vi "AlliGator Check Calibration Menu Items.vi"(8 "Use Calibration Phasor Map":bool, 9 "Use Calibration Phasor Curve":bool, 10 "Use Calibration Phasor":bool, 11 "Menu in":refnum<k9>) -> (3 "menu reference out":refnum<k9>)   [LabVIEW 2021, in "AlliGator Phasor Calibration.lvlib"]
doc: "Checks the appropriate menu item telling what type of calibration is used (single phasor, map or series)."
uses:
  AlliGator Phasor Calibration.lvlib
panel:
  # "see the AlliGator License on the block diagram (Ctrl+E or Window:Show Block Diagram)"
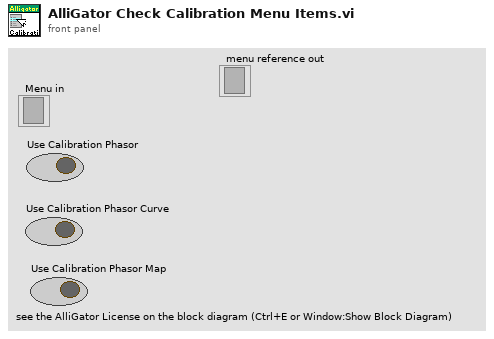
[diagram p1: front panel]
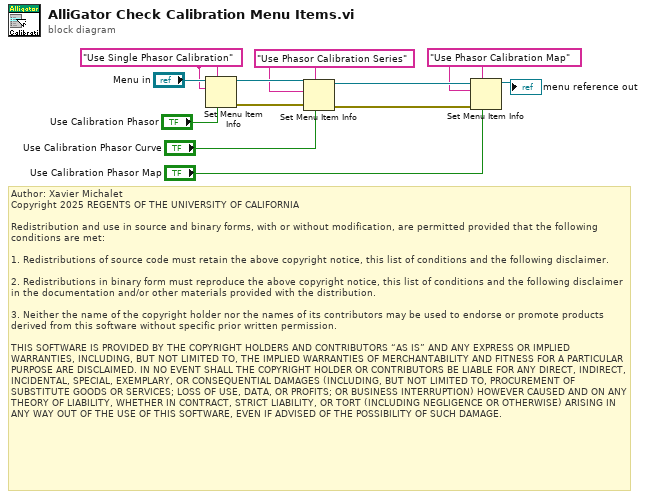
[diagram p0: block diagram]
diagram:
  w1 = "Use Phasor Calibration Map" ("item name")
  w6 = "Use Phasor Calibration Series" ("item name")
  w7 = "Use Single Phasor Calibration" ("item name")
  # "Author: Xavier Michalet\nCopyright 2025 REGENTS OF THE UNIVERSITY OF CALIFORNIA\n\nRedistribution and use in source and binary forms, with or without modification, are permitted provided that the following conditions are met:\n\n1. Redistributions of source code must retain the above copyright notice, this list of conditions and the following disclaimer.\n\n2. Redistributions in binary form must reproduce the above copyright notice, this list of conditions and the following disclaimer in the documentation and/or other materials provided with the distribution.\n\n3. Neither the name of the copyright holder nor the names of its contributors may be used to endorse or promote products derived from this software without specific prior written permission.\n\nTHIS SOFTWARE IS PROVIDED BY THE COPYRIGHT HOLDERS AND CONTRIBUTORS “AS IS” AND ANY EXPRESS OR IMPLIED WARRANTIES, INCLUDING, BUT NOT LIMITED TO, THE IMPLIED WARRANTIES OF MERCHANTABILITY AND FITNESS FOR A PARTICULAR PURPOSE ARE DISCLAIMED. IN NO EVENT SHALL THE COPYRIGHT HOLDER OR CONTRIBUTORS BE LIABLE FOR ANY DIRECT, INDIRECT, INCIDENTAL, SPECIAL, EXEMPLARY, OR CONSEQUENTIAL DAMAGES (INCLUDING, BUT NOT LIMITED TO, PROCUREMENT OF SUBSTITUTE GOODS OR SERVICES; LOSS OF USE, DATA, OR PROFITS; OR BUSINESS INTERRUPTION) HOWEVER CAUSED AND ON ANY THEORY OF LIABILITY, WHETHER IN CONTRACT, STRICT LIABILITY, OR TORT (INCLUDING NEGLIGENCE OR OTHERWISE) ARISING IN ANY WAY OUT OF THE USE OF THIS SOFTWARE, EVEN IF ADVISED OF THE POSSIBILITY OF SUCH DAMAGE."
  n1 = Set Menu Item Info(6:"Use Calibration Phasor", 7:w7, 10:w7, 11:"Menu in") -> (0:w9:errorcluster, 3:w10:refnum<k9>)  [unwired: 3 in]
  n2 = Set Menu Item Info(6:"Use Calibration Phasor Curve", 7:w6, 8:w9, 10:w6, 11:w10) -> (0:w5:errorcluster, 3:w4:refnum<k9>)  [unwired: 2 in]
  n3 = Set Menu Item Info(6:"Use Calibration Phasor Map", 7:w1, 8:w5, 10:w1, 11:w4) -> (3:→"menu reference out":refnum<k9>)  [unwired: 2 in, 1 out]
